vi "Read Config.vi"(8 "error in (no error)":errorcluster, 9 "Re-Init?":bool, 10 "ICM File In":path, 11 "Lookup Table in":refnum<class "Lookup Table.lvclass">) -> (0 "error out":errorcluster, 3 "Lookup Table out":refnum<class "Lookup Table.lvclass">)   [LabVIEW 2015, in "Lookup Table.lvclass"]
doc: "Lookup Table.lvclass:Read Config.vi\n\nThis VI reads the Lookup Table Class parameters from the ICM configuration file.\n\nInstrument Communication Module Version 1.0\nSeptember, 2017 Original Code Consulting David Thomson\n www.originalcode.com"
uses:
  Lookup Table.lvclass
  Lookup Table.lvclass/Lookup Table.ctl
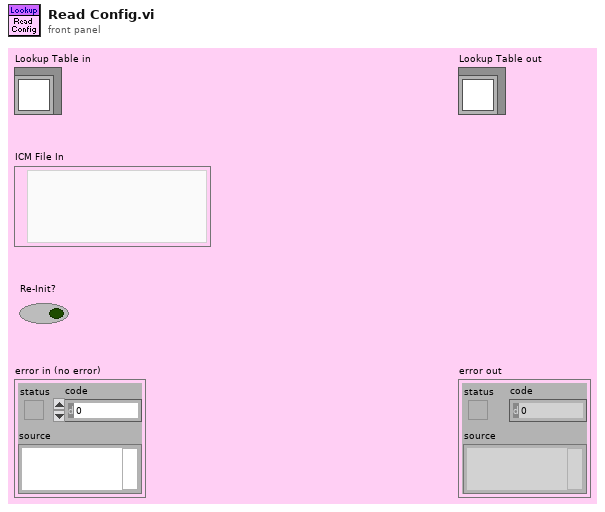
[diagram p1: front panel]
types:
  T1 = typedef "Lookup Table Config.ctl" = cluster{"Tables":cluster{"Instance":string, "Table":cluster{"Raw Value":dbl, "Sca;ed Value":dbl}[]}[]}
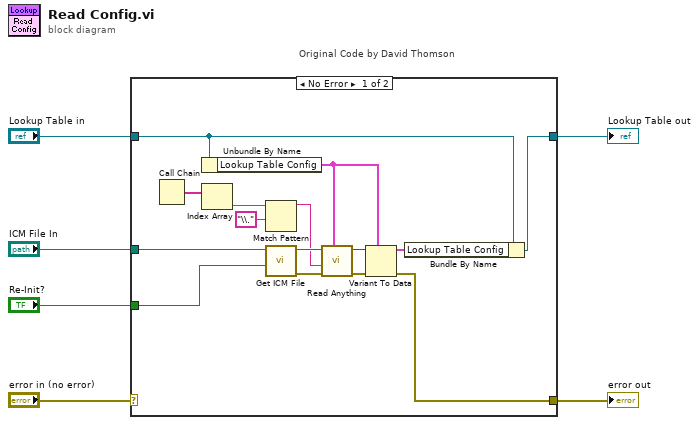
[diagram p0: block diagram]
diagram:
  n1 = case "Original Code by David Thomson" shown="No Error" "error in (no error)" {
    selector: "error in (no error)" -> [_ w23]
    tunnel: [w13 w23] -> w5
    tunnel: [w9 w22] -> w3
    tunnel: "Lookup Table in" -> [w11 w22]
    tunnel: "ICM File In" -> [w8 _]
    tunnel: "Re-Init?" -> [w7 _]
    frame No Error {
      n2 = Call Chain() -> (call chain=w18:string[])
      n3 = Unbundle By Name(w11) -> ("Lookup Table Config"=w10:T1)
      n4 = Index Array(array=w18) -> (element=w19:string)  [unwired: 1 in]
      n5 = Match Pattern(string=w19, regular expression="\\.") -> (before substring=w16:string)  [unwired: 1 in, 3 out]
      n6 = call "Get ICM File.vi"("Re-Init?"=w7, "ICM File In"=w8) -> ("error out"=w20:errorcluster, "ICM File"=w21:path)  [unwired: 8 in]
      n7 = call "Read Anything.vi"("Type of Anything"=w10, "Error In"=w20, "Section Name (Name of \"Type of Anything\")"=w16, "Path (dialog)"=w21) -> ("Error Out"=w14:errorcluster, "Anything"=w15:variant)  [unwired: 5 in, 1 out]
      n8 = Variant To Data(error in=w14, type=w10, Variant=w15) -> (data=w12:T1, error out=w13:errorcluster)
      n9 = Bundle By Name(cluster=w11, "Lookup Table Config"=w12) -> (w9:refnum<class "Lookup Table.lvclass">)
    }
    frame Error {
    }
  }
  "error out" <- w5
  "Lookup Table out" <- w3
